vi "Compressor With Cylinder.vi"() -> ()   [LabVIEW 2017]
doc: "Compressor with Cylinder \n\nThis example shows how to control a compressor, extend and retract a cylinder, and optionally use a limit switch to retract automatically.\n\nThis example works with the PCM (Pneumatic Control Module) communicating with the roboRIO over CAN bus. The PCM must also be supplied with 12V DC from the PDP (Power Distribution Panel).\n\nThe Compressor, Pressure Switch, and Solenoids are all wired to the PCM \n\nThe Limit Switch is wired to DIO 9. It causes the cylinder to retract when the Auto Retract button is pressed.\n\nRefer to the Pneumatics Manual for air connections. Your pneumatics setup should include a compressor, pressure switch, tank, regulator, valve, flow controls, cylinder, plug valve, etc.\n\nTo run this example you should have a pneumatic system with air pressure connected to the P input on the SMC double solenoid valve. The A output of the valve should be connected via a flow control to the backend of a cylinder. The B output of the valve should be connected via a flow control to the frontend of a cylinder. When the cylinder is extended, it should physically depress the Limit Switch.\n\nWith the VI running, pressing the Extend button will push the cylinder shaft out, and pressing the Retract button will pull it back. Notice that the Extend and Retract buttons have their Mechanical Action set to Latch When Pressed. This means they stay pressed (ON) until they are read by the program, then they return to the OFF position. This works because once the SMC solenoid valve is pulled one direction, it stays in that position until it is pulled in the opposite direction - it only needs to be momentarily energized. The Auto Retract button can be used to make the cylinder return automatically. With the Auto Retract button ON, pressing the Extend button will push the cylinder out, and it will retract when it hits the limit switch.\n\nThis example expects a USB cable connected from your development PC to the Type B USB Jack (next to the power input) on the roboRIO.\n\nThis example expects the Driver Station to be running."
uses:
  <vilib>/Rock Robotics/WPI/Solenoid/WPI_SolenoidChannel.ctl
  <vilib>/Rock Robotics/SystemInterfaces/DIO/FPGA_DIOChannel.ctl
  <vilib>/Rock Robotics/WPI/Solenoid/WPI_SolenoidValue.ctl
  <vilib>/Rock Robotics/WPI/Solenoid/WPI_SolenoidOpenDouble.vi
  <vilib>/Rock Robotics/WPI/Solenoid/WPI_SolenoidSetEnum.vi
panel:
  out "Compressor Running":bool
  out "Cylinder Limit":bool
  in  "Limit Switch Channel":T1=enum."DIO 9"
  in  "Auto Retract":bool
  in  "Retract":bool
  in  "Retract Solenoid Channel":T2
  in  "Extend Solenoid Channel":T2=enum."Solenoid 1"
  out "Compressor Monitoring":bool
  in  "stop":bool
  in  "Extend":bool
  # "Set these inputs before running."
  # "roboRIO Wiring Diagram"
  # "when extended, the cylinder should depress this"
  # "Limit\nSwitch"
  # "These can be set while running."
  # "Pneumatic Control Module Wiring Diagram"
  # "Output information."
  # "Connect\nPower in\nHere"
  # "Connect\nCompressor\nHere"
  # "tubing port for retract side of cylinder"
  # "tubing port for extend side of cylinder"
  # "Pressure\nSwitch"
  # "SMC double solenoid valve"
  # "CAN"
  # "COMPRESSOR OUT"
  # "PRESSURE"
  # "NC"
  # "C"
  # "B"
  # "A"
  # "B"
  # "A"
  # "COM"
  # "NC"
  # "NO"
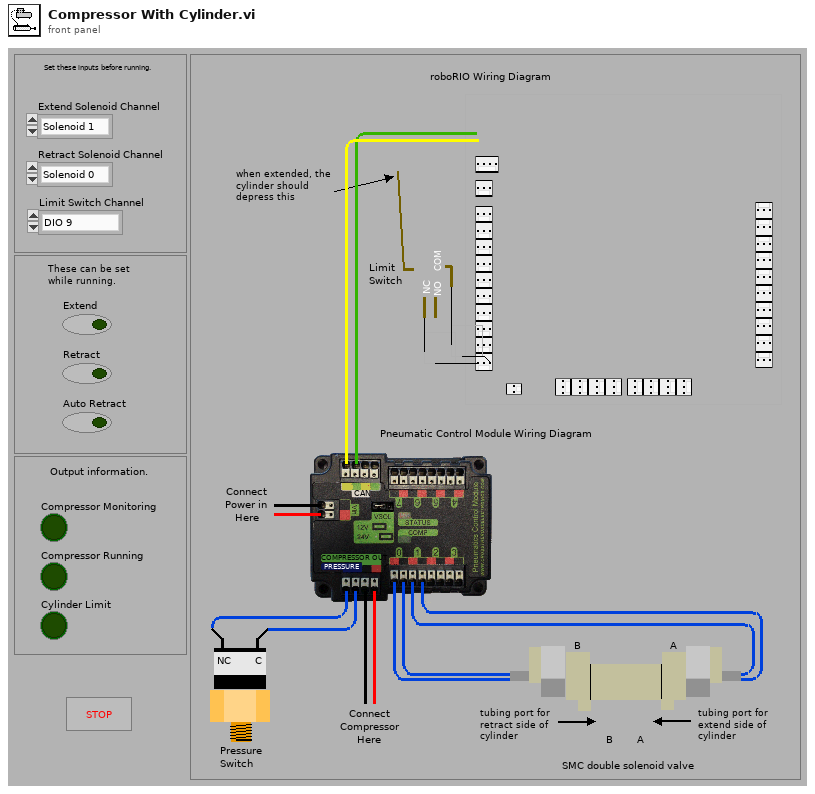
[diagram p1: front panel]
types:
  T1 = typedef "FPGA_DIOChannel.ctl" = enum8{"DIO 0", "DIO 1", "DIO 2", "DIO 3", "DIO 4", "DIO 5", "DIO 6", "DIO 7", "DIO 8", "DIO 9", "DIO MXP 0", "DIO MXP 1", "DIO MXP 2", "DIO MXP 3", "DIO MXP 4", "DIO MXP 5", "DIO MXP 6", "DIO MXP 7", "DIO MXP 8", "DIO MXP 9", "DIO MXP 10", "DIO MXP 11", "DIO MXP 12", "DIO MXP 13", "DIO MXP 14", "DIO MXP 15", "SPI Port CS1", "SPI Port CS2", "SPI Port CS3", "SPI Port MISO", "SPI Port MOSI", "Invalid"}
  T2 = typedef "WPI_SolenoidChannel.ctl" = enum8{"Solenoid 0", "Solenoid 1", "Solenoid 2", "Solenoid 3", "Solenoid 4", "Solenoid 5", "Solenoid 6", "Solenoid 7", "Invalid"}
  T3 = typedef "WPI_CompressorDevRef.ctl" = cluster{"DevStatus":errorcluster, "Pneumatics Control Module":u8}
  T4 = typedef "WPI_DigitalInputDevRef.ctl" = cluster{"DevStatus":errorcluster, "DIO Channel":T1}
  T5 = typedef "WPI_SolenoidDevRef.ctl" = cluster{"DevStatus":errorcluster, "Pneumatics Control Module":u8, "Forward Solenoid Channel":T2, "Reverse Solenoid Channel":T2}
  T6 = typedef "WPI_SolenoidValue.ctl" = enum16{"Off", "On", "Forward", "Reverse"}
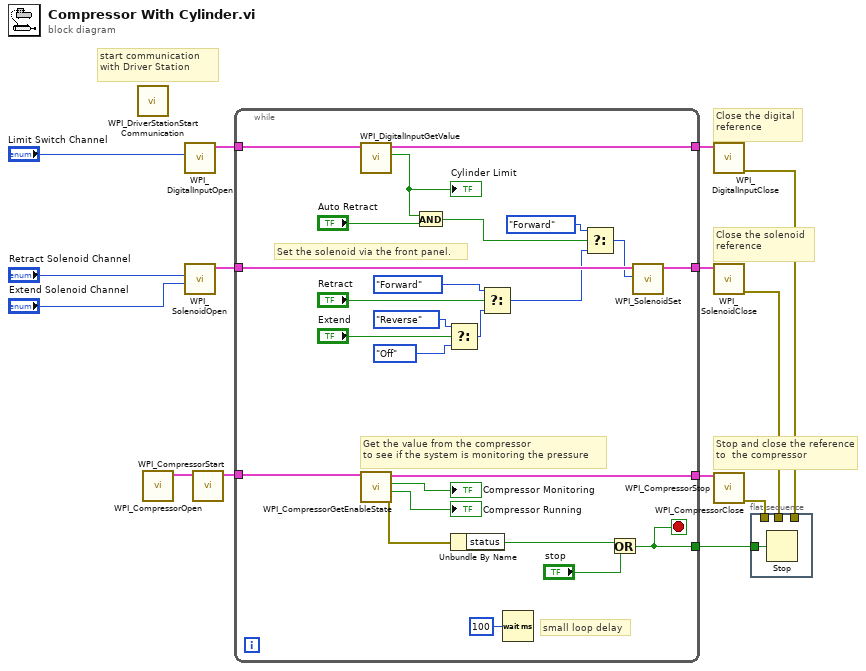
[diagram p0: block diagram]
diagram:
  # "Close the digital\nreference"
  # "Close the solenoid\nreference"
  # "start communication with Driver Station"
  # "Stop and close the reference to  the compressor"
  n1 = call <vilib>:"WPI_DriverStationStart Communication.vi"() -> ()  [unwired: 2 in, 10 out]
  n2 = call <vilib>:"WPI_CompressorOpen.vi"() -> ("CompressorDevRef"=w5:T3)  [unwired: 14 in, 1 out]
  n3 = call <vilib>:"WPI_DigitalInputOpen.vi"("DIO Channel"="Limit Switch Channel") -> ("DigitalInputDevRef"=w9:T4)  [unwired: 1 in, 9 out]
  n4 = call-poly <vilib>:"WPI_SolenoidOpen.vi"("Reverse Solenoid Channel"="Extend Solenoid Channel", "Forward Solenoid Channel"="Retract Solenoid Channel") -> ("SolenoidDevRef"=w11:T5)  [unwired: 2 in, 7 out]
  n5 = call <vilib>:"WPI_CompressorStart.vi"("CompressorDevRef"=w5) -> ("CompressorDevRef"=w14:T3)  [unwired: 1 in, 9 out]
  n6 = while {
    tunnel: w14 -> [w40]
    tunnel: [w39] -> w13
    tunnel: [w37] -> w4
    tunnel: w11 -> [w32]
    tunnel: [w22] -> w12
    tunnel: w9 -> [w31]
    tunnel: [w30] -> w8
    stop <- w37 stop-if-true
    # "small loop delay"
    # "Get the value from the compressor \nto see if the system is monitoring the pressure"
    # "Set the solenoid via the front panel."
    n7 = call <vilib>:"WPI_DigitalInputGetValue.vi"("DigitalInputDevRef"=w31) -> ("Value"=w20:bool, "DigitalInputDevRef"=w30:T4)  [unwired: 1 in, 8 out]
    "Cylinder Limit" <- w20
    n8 = call <vilib>:"WPI_CompressorGetEnableState.vi"("CompressorDevRef"=w40) -> ("error out"=w35:errorcluster, "Compressor Running"=→"Compressor Running":bool, "Enabled"=→"Compressor Monitoring":bool, "CompressorDevRef"=w39:T3)  [unwired: 1 in, 6 out]
    n9 = And(x=w20, y="Auto Retract") -> (x .and. y?=w16:bool)
    n10 = Select(t=WPI_SolenoidValue."Reverse" ("Value"), s="Extend", f=WPI_SolenoidValue."Off" ("Value")) -> (s? t:f=w24:T6)
    n11 = Unbundle By Name(w35) -> ("status"=w34:bool)
    n12 = Select(t=WPI_SolenoidValue."Forward" ("Value"), s="Retract", f=w24) -> (s? t:f=w17:T6)
    n13 = Wait (ms)(milliseconds to wait=u32 100) -> ()  [unwired: 1 out]
    n14 = Select(t=WPI_SolenoidValue."Forward" ("Value"), s=w16, f=w17) -> (s? t:f=w18:T6)
    n15 = Or(x=w34, y="stop") -> (x .or. y?=w37:bool)
    n16 = call-poly <vilib>:"WPI_SolenoidSet.vi"("Value"=w18, "SolenoidDevRef"=w32) -> ("SolenoidDevRef"=w22:T5)  [unwired: 1 in, 8 out]
  }
  n17 = call <vilib>:"WPI_DigitalInputClose.vi"("DigitalInputDevRef"=w8) -> ("error out"=w1:errorcluster)  [unwired: 1 in, 9 out]
  n18 = call <vilib>:"WPI_SolenoidClose.vi"("SolenoidDevRef"=w12) -> ("error out"=w2:errorcluster)  [unwired: 1 in, 9 out]
  n19 = call <vilib>:"WPI_CompressorStop.vi"("CompressorDevRef"=w13) -> ("CompressorDevRef"=w15:T3)  [unwired: 1 in, 9 out]
  n20 = call <vilib>:"WPI_CompressorClose.vi"("CompressorDevRef"=w15) -> ("error out"=w3:errorcluster)  [unwired: 1 in, 9 out]
  n21 = flat-sequence {
    tunnel: w4 -> [w41]
    tunnel: w3 -> [_]
    tunnel: w2 -> [_]
    tunnel: w1 -> [_]
    frame #0 {
      n22 = Stop(stop? (T)=w41) -> ()
    }
  }
